vi "ErrorCountUpdated.vi"(8 "error in (no error)":errorcluster, 10 "ErrorCount":u32, 11 "TCP_Server in":refnum<class "TCP_Server.lvclass">) -> (0 "error out":errorcluster, 3 "TCP_Server out":refnum<class "TCP_Server.lvclass">)   [LabVIEW 2023, in "TCP_Server.lvlib" / "TCP_Server.lvclass"]
uses:
  TCP_Server.lvclass
  TCP_Server.lvclass/TCP_Server.ctl
  TCP_serverGUI/TCP_serverGUI Messages/UpdateNumberOfErrors Msg/UpdateNumberOfErrors Msg.lvclass
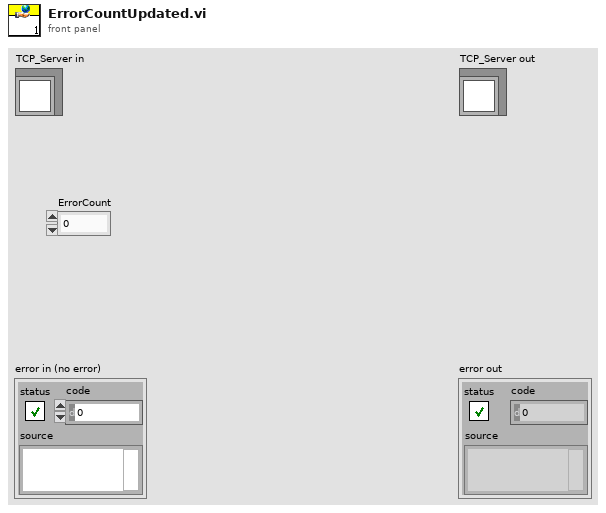
[diagram p1: front panel]
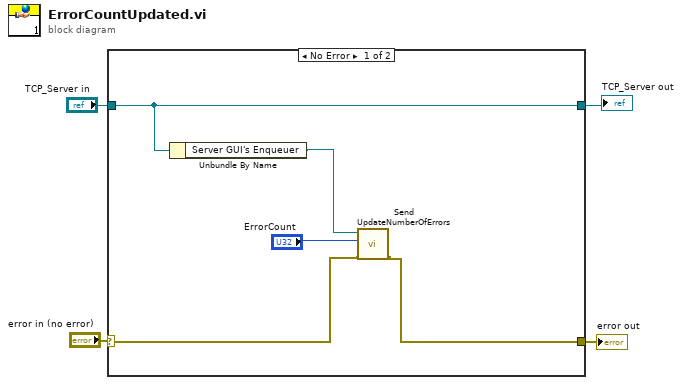
[diagram p0: block diagram]
diagram:
  n1 = case shown="No Error" "error in (no error)" {
    selector: "error in (no error)" -> [w8 w11]
    tunnel: [w7 w11] -> w3
    tunnel: "TCP_Server in" -> [w5 w10]
    tunnel: [w5 w10] -> w1
    frame No Error {
      n2 = Unbundle By Name(w5) -> ("Server GUI's Enqueuer"=w9:refnum<class "Message Enqueuer.lvclass">)
      n3 = call "Send UpdateNumberOfErrors.vi"("error in (no error)"=w8, "NumberOfErrord"="ErrorCount", "Message Enqueuer"=w9) -> ("error out"=w7:errorcluster)  [unwired: 7 in, 1 out]
    }
    frame Error {
    }
  }
  "error out" <- w3
  "TCP_Server out" <- w1
